vi "Intensity Graph to XY Graph.vi"() -> ()   [LabVIEW 2019]
uses:
  graph_utilities.lvclass
panel:
  in  "OK":bool
  out "Horizontal":cluster{dbl[], dbl[]}[](graph)
  out "Vertical":cluster{dbl[], dbl[]}[](graph)
  in  "V2f":dbl[][](graph)=array73x221[16133 elements]
  # "Control Graph:"
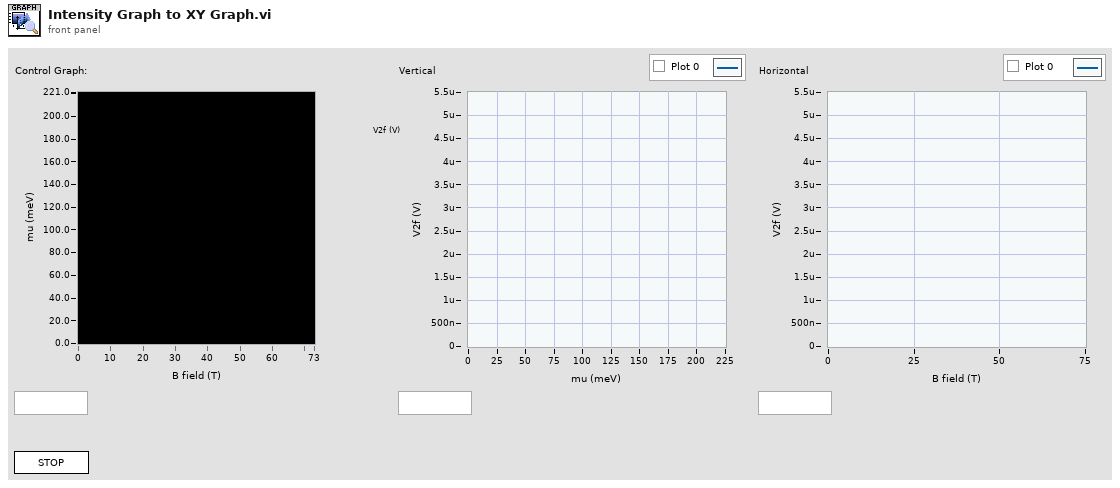
[diagram p1: front panel]
types:
  T1 = enum32{"Invalid", "Standard", "Closed", "Hidden", "Minimized", "Maximized"}
  T2 = enum32{"invalid app kind", "Development System", "Run Time System", "Student Edition", "Embedded LabVIEW", "Evaluation", "Custom"}
  T3 = cluster{"Core":cluster{"Current VI Reference":refnum<vi>, "Close Panel on Exit?":bool}, "graphs":refnum<class "graph_utilities.lvclass">[]}
  T4 = cluster{"Current VI Reference":refnum<vi>, "Close Panel on Exit?":bool}
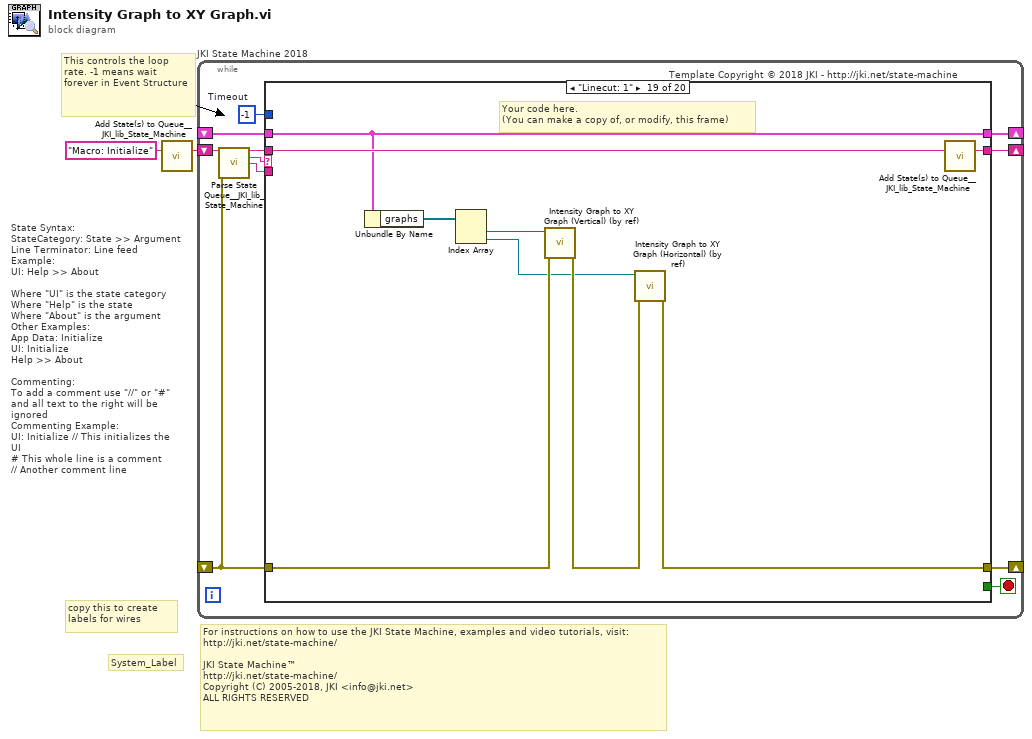
[diagram p0: block diagram]
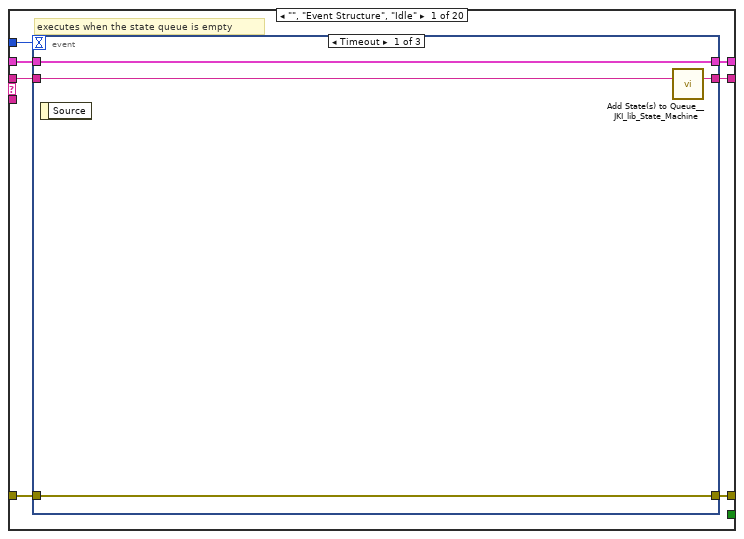
[diagram p2: hidden frame]
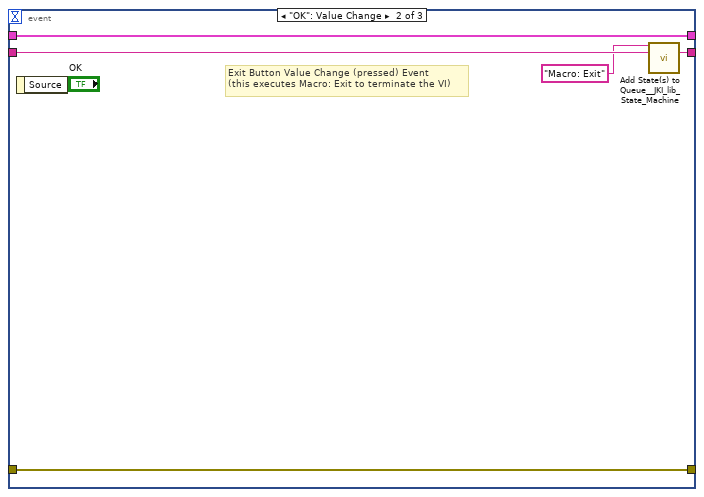
[diagram p3: hidden frame]
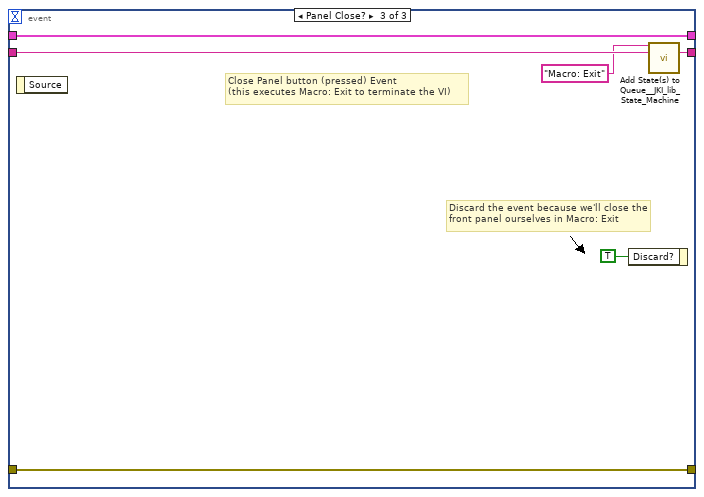
[diagram p4: hidden frame]
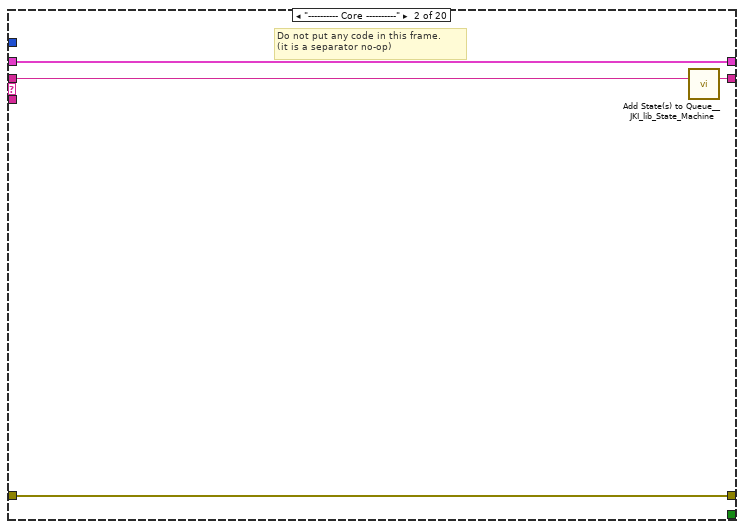
[diagram p5: hidden frame]
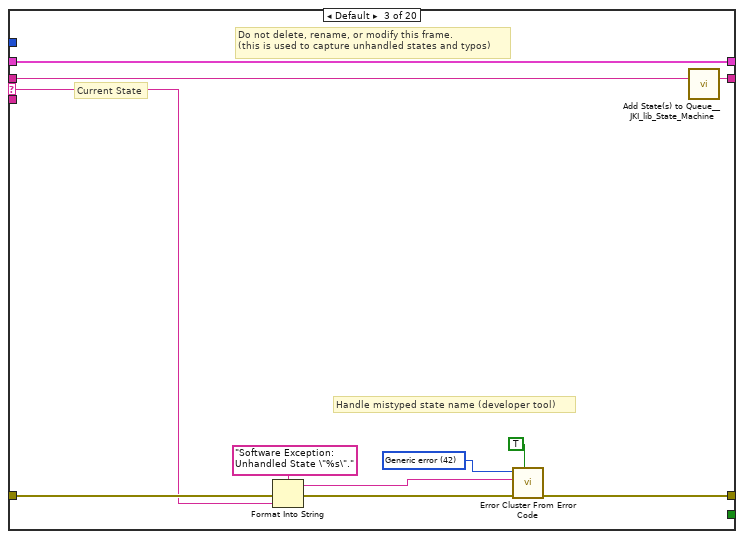
[diagram p6: hidden frame]
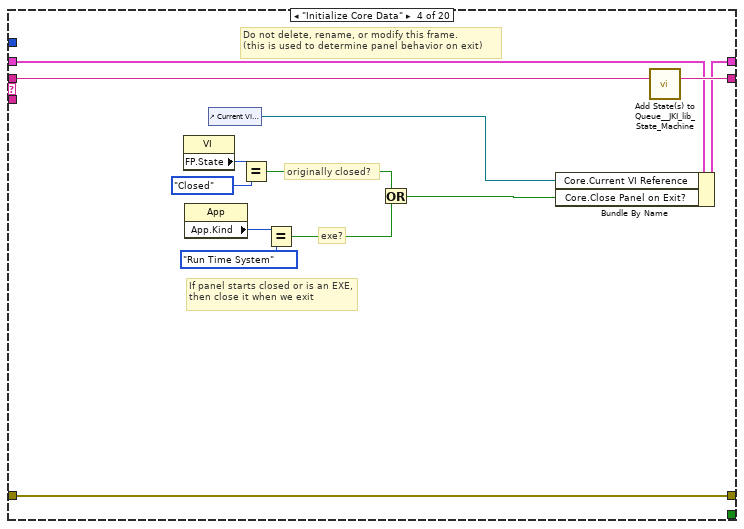
[diagram p7: hidden frame]
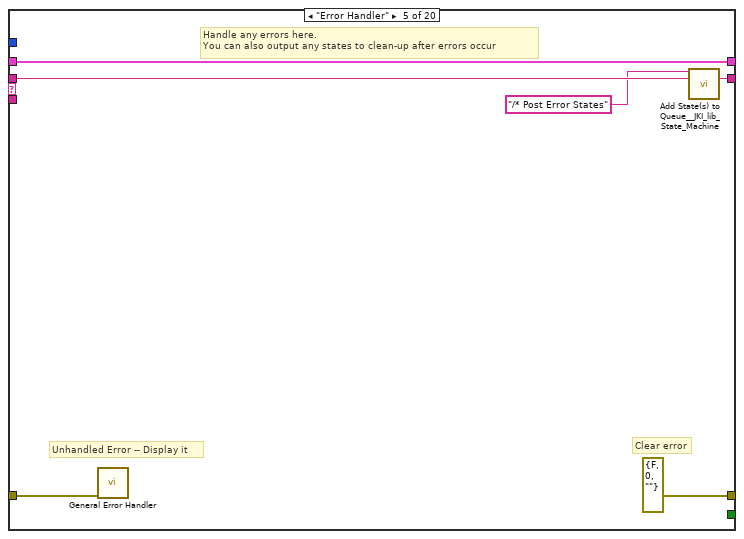
[diagram p8: hidden frame]
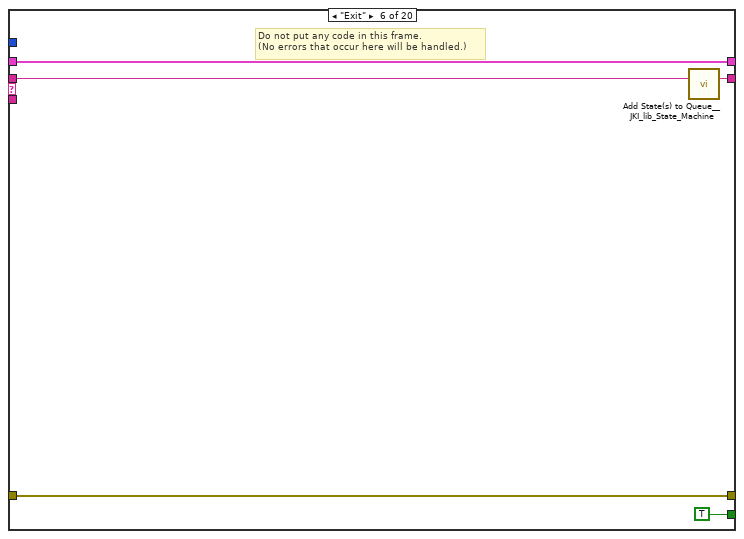
[diagram p9: hidden frame]
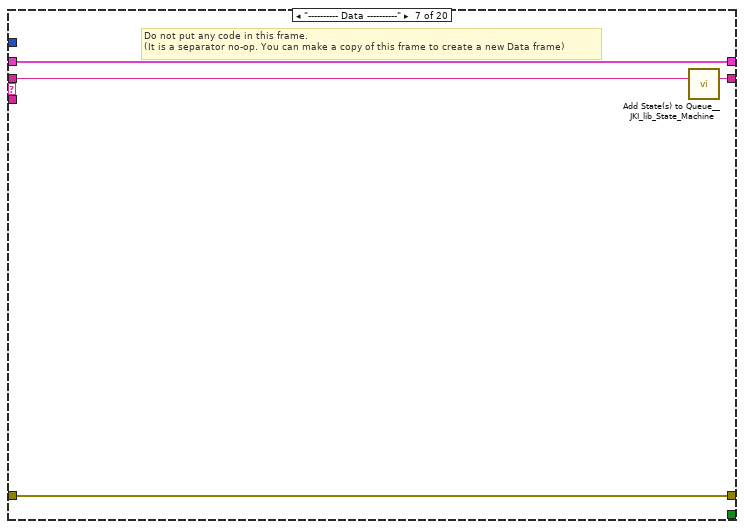
[diagram p10: hidden frame]
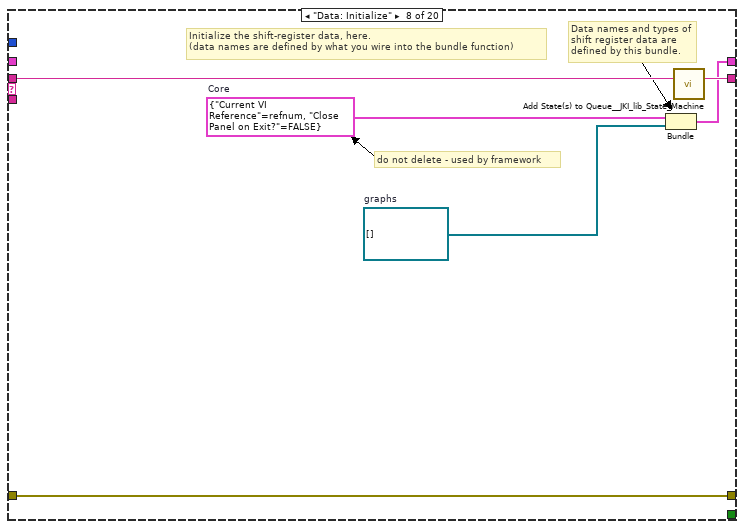
[diagram p11: hidden frame]
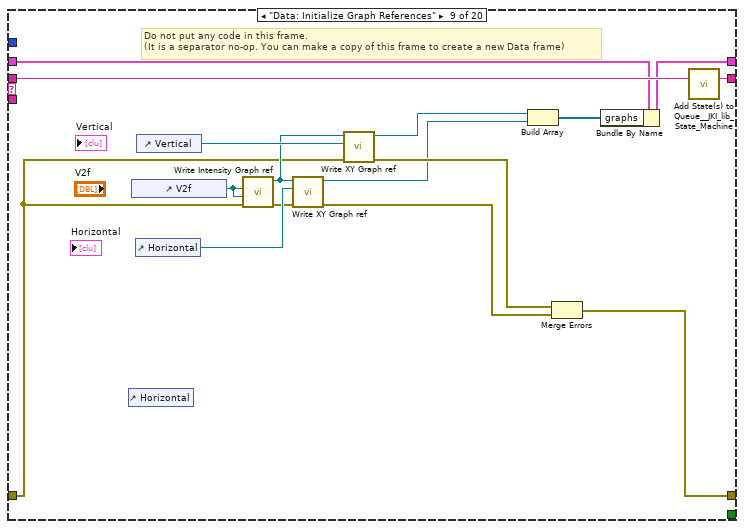
[diagram p12: hidden frame]
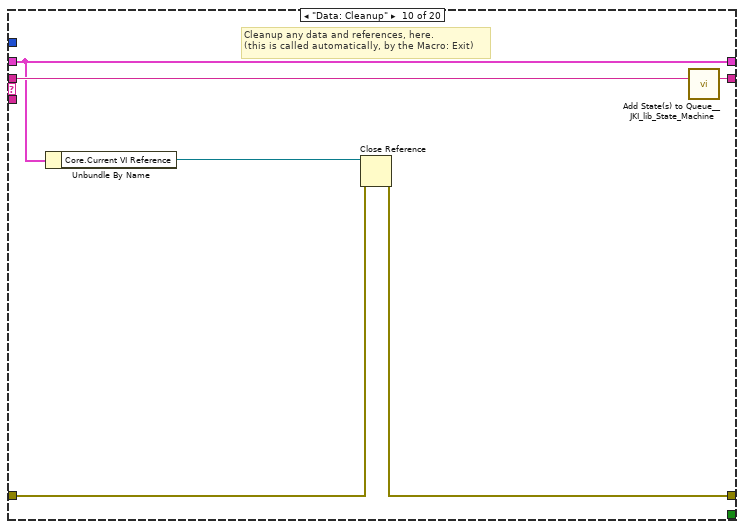
[diagram p13: hidden frame]
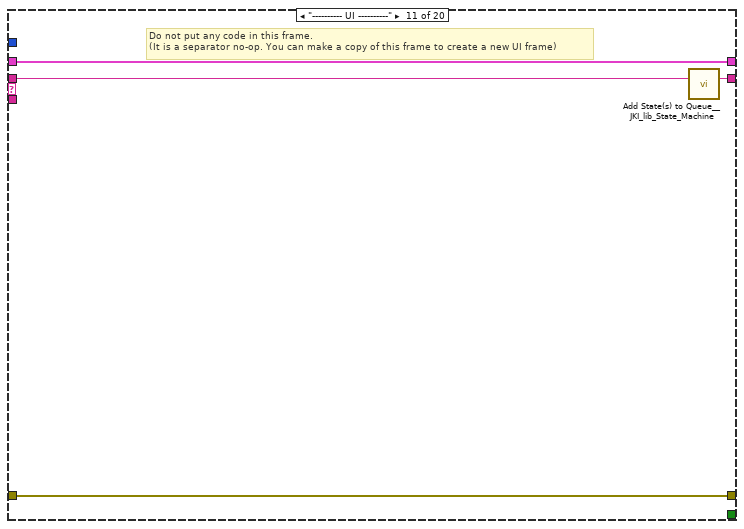
[diagram p14: hidden frame]
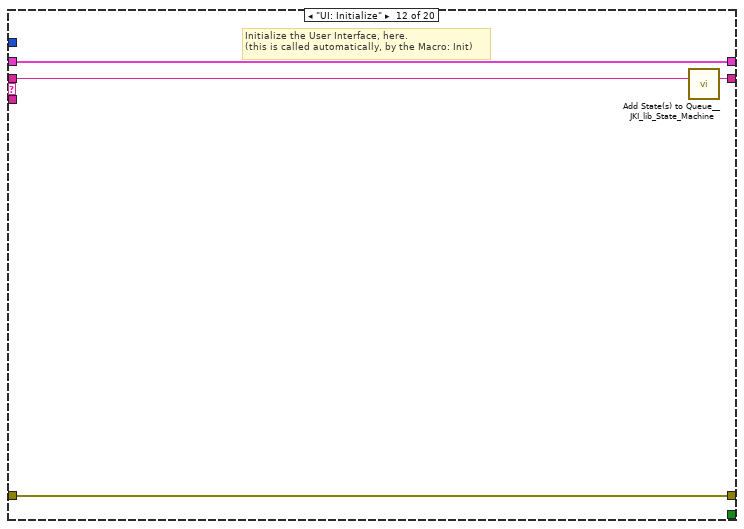
[diagram p15: hidden frame]
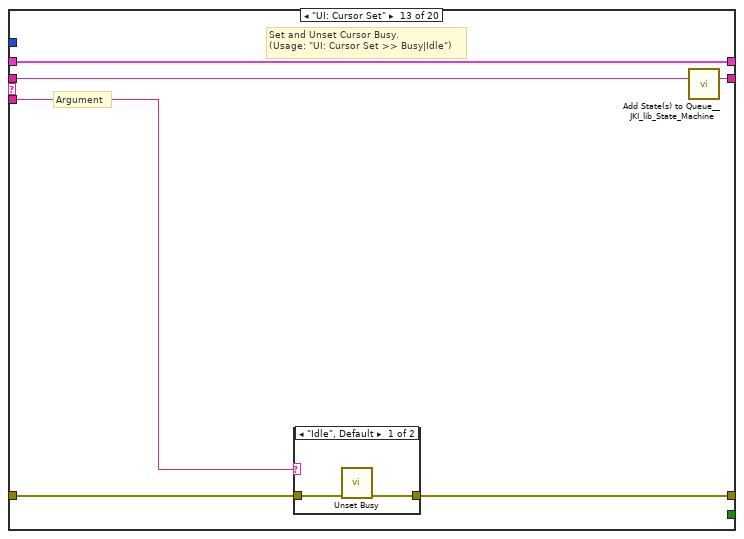
[diagram p16: hidden frame]
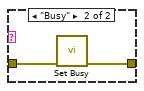
[diagram p17: hidden frame]
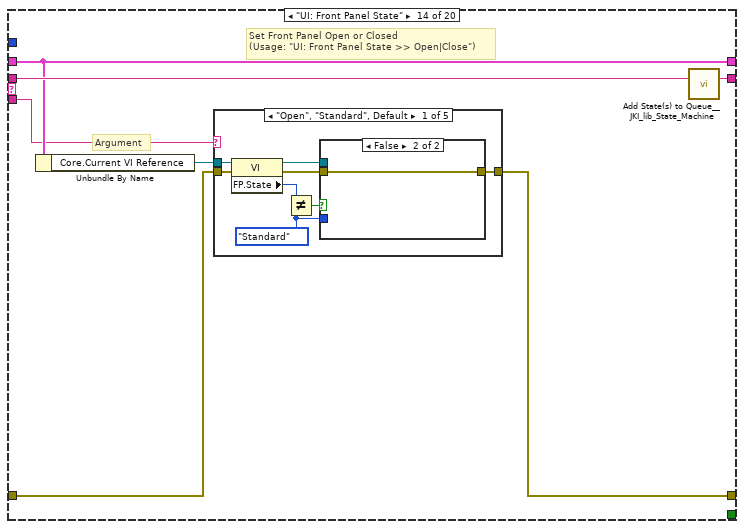
[diagram p18: hidden frame]
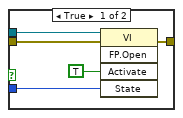
[diagram p19: hidden frame]
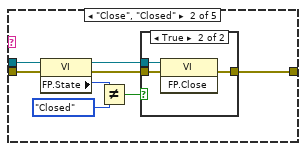
[diagram p20: hidden frame]
diagram:
  # "For instructions on how to use the JKI State Machine, examples and video tutorials, visit:\nhttp://jki.net/state-machine/\n\nJKI State Machine™\nhttp://jki.net/state-machine/\nCopyright (C) 2005-2018, JKI <info@jki.net>\nALL RIGHTS RESERVED"
  # "State Syntax:\nStateCategory: State >> Argument\nLine Terminator: Line feed\nExample:\nUI: Help >> About\n\nWhere \"UI\" is the state category\nWhere \"Help\" is the state\nWhere \"About\" is the argument\nOther Examples:\nApp Data: Initialize\nUI: Initialize\nHelp >> About\n\nCommenting:\nTo add a comment use \"//\" or \"#\" and all text to the right will be ignored\nCommenting Example:\nUI: Initialize // This initializes the UI\n# This whole line is a comment\n// Another comment line"
  # "copy this to create labels for wires"
  # "This controls the loop rate. -1 means wait forever in Event Structure"
  # "System_Label"
  n1 = call <vilib>:"Add State(s) to Queue__JKI_lib_State_Machine.vi"("State(s) in (\"\")"="Macro: Initialize") -> ("States Out"=w2:string)  [unwired: 14 in]
  n2 = while "JKI State Machine 2018" {
    shift-right: [w6] -> _
    shift-left: _ -> [w5]
    shift-right: [w9] -> _
    shift-left: _ -> [w3]
    shift-right: [w8] -> _
    shift-left: w2 -> [w10]
    stop <- w7 stop-if-true
    w4 = -1  # Timeout
    # "Template Copyright © 2018 JKI - http://jki.net/state-machine"
    n3 = call <vilib>:"Parse State Queue__JKI_lib_State_Machine.vi"("State Queue"=w10, "Error In (no error)"=w3) -> ("Remaining States"=w12:string, "Current State"=w13:string, "Arguments"=w11:string)  [unwired: 11 in]
    n4 = case shown="\"Linecut: 1\"" w13 {
      selector: w13 -> [_ _ w40 _ _ _ _ _ _ _ _ _ _ _ _ _ _ _ _ _]
      tunnel: w12 -> [w20 w39 w44 w63 w69 w74 w78 w84 w100 w106 w110 w114 w120 w131 w200 w206 w216 w220 w229 w233]
      tunnel: w11 -> [_ _ _ _ _ _ _ _ _ _ _ _ w115 w125 _ _ _ _ _ _]
      tunnel: w5 -> [w18 w36 w42 w56 w66 w72 w75 _ w91 w101 w107 w112 w118 w127 w197 w203 w213 w217 w227 w230]
      tunnel: [w17 w37 w46 w60 errorcluster {"status"=FALSE, "code"=0, "source"=""} ("error out") w71 w76 w81 w86 w102 w108 w111 w116 w128 w198 w204 w214 w218 w222 w231] -> w9
      tunnel: w3 -> [w16 w37 w45 w60 w65 w71 w76 w81 w85 w103 w108 w111 w117 w129 w198 w204 w214 w218 w224 w231]
      tunnel: [w19 w38 w43 w62 w68 w73 w77 w83 w99 w105 w109 w113 w119 w130 w199 w205 w215 w219 w228 w232] -> w8
      tunnel: [_ _ _ _ _ TRUE _ _ _ _ _ _ _ _ _ _ _ _ _ _] -> w7
      tunnel: [w15 w36 w42 w61 w66 w72 w75 w82 w90 w101 w107 w112 w118 w127 w197 w203 w213 w217 w227 w230] -> w6
      tunnel: w4 -> [w14 _ _ _ _ _ _ _ _ _ _ _ _ _ _ _ _ _ _ _]
      frame "", "Event Structure", "Idle" {
        # "executes when the state queue is empty"
        n5 = event shown="[0] Timeout" {
          selector: _ -> [_ _ _]
          dyn-events: _ -> [_ _ _]
          timeout: w14 -> [_ _ _]
          tunnel: w20 -> [w24 w29 w35]
          tunnel: [w23 w28 w34] -> w19
          tunnel: w18 -> [w21 w26 w32]
          tunnel: [w22 w27 w33] -> w17
          tunnel: w16 -> [w22 w27 w33]
          tunnel: [w21 w26 w32] -> w15
          event Timeout {
            n6 = event-data() -> ()  [unwired: 1 in, 1 out]
            n7 = call <vilib>:"Add State(s) to Queue__JKI_lib_State_Machine.vi"("State(s) in (\"\")"=w24) -> ("States Out"=w23:string)  [unwired: 14 in]
          }
          event "OK": Value Change {
            # "Exit Button Value Change (pressed) Event\n(this executes Macro: Exit to terminate the VI)"
            n8 = event-data() -> ()  [unwired: 1 in, 1 out]
            n9 = call <vilib>:"Add State(s) to Queue__JKI_lib_State_Machine.vi"("State(s) in Front (\"\")"="Macro: Exit", "State(s) in (\"\")"=w29) -> ("States Out"=w28:string)  [unwired: 13 in]
          }
          event Panel Close? {
            # "Discard the event because we'll close the front panel ourselves in Macro: Exit"
            # "Close Panel button (pressed) Event\n(this executes Macro: Exit to terminate the VI)"
            n10 = event-data() -> ()  [unwired: 1 in, 1 out]
            n11 = event-data("Discard?"=TRUE) -> ()  [unwired: 1 in, 1 out]
            n12 = call <vilib>:"Add State(s) to Queue__JKI_lib_State_Machine.vi"("State(s) in Front (\"\")"="Macro: Exit", "State(s) in (\"\")"=w35) -> ("States Out"=w34:string)  [unwired: 13 in]
          }
        }
      }
      frame "---------- Core ----------" {
        # "Do not put any code in this frame.\n(it is a separator no-op)"
        n13 = call <vilib>:"Add State(s) to Queue__JKI_lib_State_Machine.vi"("State(s) in (\"\")"=w39) -> ("States Out"=w38:string)  [unwired: 14 in]
      }
      frame Default {
        w49 = 42 items=["No error", "Argument error", "Memory is full", "Out of zone", "End of file", "File already open", "Generic file I/O error", "File not found", "File permission error", "Disk is full", "Duplicate path", "Too many files open", "System feature not enabled", "Resource file not found", "Cannot add resource", "Resource not found", "Image not found", "Image memory error", "Pen does not exist", "Config type invalid", "Config token not found", "Config parse error", "Config memory error", "Bad external code format", "Bad external code offset", "External code not present", "Null window", "Destroy window error", "Null menu", "Print aborted", "Bad print record", "Print driver error", "Windows error during printing", "Memory error during printing", "Print dialog error", "Generic print error", "Invalid device refnum", "Device not found", "Device parameter error", "Device unit error", "Cannot open device", "Device call aborted", "Generic error", "Cancelled by user", "Object ID too low", "Object ID too high", "Object not in heap", "Unknown heap", "Unknown object (invalid DefProc)", "Unknown object (DefProc not in table)", "Message out of range", "Invalid (null) method", "Unknown message", "Manager call not supported", "Bad address", "Network operation in progress", "Network operation timed out", "Connection is busy", "Network attribute not supported", "Network error", "Address in use", "System out of memory", "Connection aborted", "Connection refused", "Not connected", "Already connected", "Connection closed", "Initialization error (interapplication manager)", "Bad occurrence", "Wait on unbound occurrence handler", "Occurrence queue overflow", "Datalog type conflict", "Unused", "Unrecognized type (interapplication manager)", "Memory corrupt", "Failed to make temporary DLL", "Old CIN version", "Drag socket not found", "Failed to load drop-object", "Failed to register OLE object", "Failed to release OLE object", "Format specifier type mismatch", "Unknown format specifier", "Too few format specifiers", "Too many format specifiers", "Scan failed", "Newer CIN version", "Error converting to variant", "Runtime menu error", "Password tampered", "Variant attribute not found", "Incompatible variant data type", "Event data is not available", "Event Store is not present", "Occurrence is not found", "Event Queue is not created", "Event info is not available", "Refnum passed is NULL", "Error retrieving Class GUID", "Error retrieving CoClass GUID", "Error retrieving TypeLib GUID.", "Bad built application magic bytes.", "Specific driver is different from the specific driver associated with the Logical Name.", "There is no session opened to the class driver.", "Max Error", "MAX - Error with config objects", "MAX - Error loading configuration", "MAX - Group not supported"]
        # "Current State"
        # "Do not delete, rename, or modify this frame.\n(this is used to capture unhandled states and typos)"
        # "Handle mistyped state name (developer tool)"
        n14 = Format Into String(format string="Software Exception: Unhandled State \"%s\"." ("message"), error in=w45, w40) -> (resulting string=w48:string, error out=w47:errorcluster)  [unwired: 1 in]
        n15 = call <vilib>:"Error Cluster From Error Code.vi"("show call chain? (False)"=TRUE, "error in (no error)"=w47, "error message (\"\")"=w48, "error code (0)"=w49) -> ("error out"=w46:errorcluster)  [unwired: 5 in]
        n16 = call <vilib>:"Add State(s) to Queue__JKI_lib_State_Machine.vi"("State(s) in (\"\")"=w44) -> ("States Out"=w43:string)  [unwired: 14 in]
      }
      frame "Initialize Core Data" {
        # "Do not delete, rename, or modify this frame.\n(this is used to determine panel behavior on exit)"
        # "originally closed?"
        # "exe?"
        # "If panel starts closed or is an EXE, then close it when we exit"
        n17 = property class="VI"() -> ("FP.State"=w53:T1)  [unwired: 2 in, 2 out]
        n18 = property class="App"() -> ("App.Kind"=w59:T2)  [unwired: 2 in, 2 out]
        n19 = control-ref of="Current VI Reference"() -> (w54:refnum<vi>)
        n20 = Equal?(x=w53, y=T1."Closed" ("Front Panel Window:State")) -> (x = y?=w51:bool)
        n21 = Equal?(x=w59, y=T2."Run Time System" ("Application:Kind")) -> (x = y?=w57:bool)
        n22 = Or(x=w51, y=w57) -> (x .or. y?=w55:bool)
        n23 = Bundle By Name(cluster=w56, "Core.Current VI Reference"=w54, "Core.Close Panel on Exit?"=w55) -> (w61:T3)
        n24 = call <vilib>:"Add State(s) to Queue__JKI_lib_State_Machine.vi"("State(s) in (\"\")"=w63) -> ("States Out"=w62:string)  [unwired: 14 in]
      }
      frame "Error Handler" {
        # "Unhandled Error -- Display it"
        # "Handle any errors here.\nYou can also output any states to clean-up after errors occur"
        # "Clear error"
        n25 = call <vilib>:"General Error Handler.vi"("error in (no error)"=w65) -> ()  [unwired: 10 in, 5 out]
        n26 = call <vilib>:"Add State(s) to Queue__JKI_lib_State_Machine.vi"("State(s) in Front (\"\")"="/* Post Error States", "State(s) in (\"\")"=w69) -> ("States Out"=w68:string)  [unwired: 13 in]
      }
      frame "Exit" {
        # "Do not put any code in this frame.\n(No errors that occur here will be handled.)"
        n27 = call <vilib>:"Add State(s) to Queue__JKI_lib_State_Machine.vi"("State(s) in (\"\")"=w74) -> ("States Out"=w73:string)  [unwired: 14 in]
      }
      frame "---------- Data ----------" {
        # "Do not put any code in this frame.\n(It is a separator no-op. You can make a copy of this frame to create a new Data frame)"
        n28 = call <vilib>:"Add State(s) to Queue__JKI_lib_State_Machine.vi"("State(s) in (\"\")"=w78) -> ("States Out"=w77:string)  [unwired: 14 in]
      }
      frame "Data: Initialize" {
        w79 = refnum<class "graph_utilities.lvclass">[] []  # graphs
        w80 = T4 {"Current VI Reference"=refnum, "Close Panel on Exit?"=FALSE}  # Core
        # "do not delete - used by framework"
        # "Data names and types of shift register data are defined by this bundle."
        # "Initialize the shift-register data, here.\n(data names are defined by what you wire into the bundle function)"
        n29 = Bundle("Core"=w80, "graphs"=w79) -> (w82:T3)  [unwired: 1 in]
        n30 = call <vilib>:"Add State(s) to Queue__JKI_lib_State_Machine.vi"("State(s) in (\"\")"=w84) -> ("States Out"=w83:string)  [unwired: 14 in]
      }
      frame "Data: Initialize Graph References" {
        # "Do not put any code in this frame.\n(It is a separator no-op. You can make a copy of this frame to create a new Data frame)"
        n31 = control-ref of="Horizontal"() -> ()  [unwired: 1 out]
        n32 = control-ref of="V2f"() -> (w94:refnum<vi>)
        n33 = control-ref of="Horizontal"() -> (w96:refnum<vi>)
        n34 = control-ref of="Vertical"() -> (w98:refnum<vi>)
        n35 = call "Write Intensity Graph ref.vi"("error in (no error)"=w85, "Intensity Graph (Control)"=w94, "Intensity Graph"=w94) -> ("error out"=w95:errorcluster, "graph_utilities out"=w97:refnum<class "graph_utilities.lvclass">)  [unwired: 7 in]
        n36 = call "Write XY Graph ref.vi"("error in (no error)"=w95, "XY Graph"=w96, "graph_utilities in"=w97) -> ("error out"=w93:errorcluster, "graph_utilities out"=w88:refnum<class "graph_utilities.lvclass">)  [unwired: 7 in]
        n37 = call "Write XY Graph ref.vi"("error in (no error)"=w85, "XY Graph"=w98, "graph_utilities in"=w97) -> ("error out"=w92:errorcluster, "graph_utilities out"=w89:refnum<class "graph_utilities.lvclass">)  [unwired: 7 in]
        n38 = Build Array(w89, w88) -> (w87:refnum<class "graph_utilities.lvclass">[])
        n39 = Merge Errors(w92, w93) -> (w86:errorcluster)
        n40 = Bundle By Name(cluster=w91, "graphs"=w87) -> (w90:T3)
        n41 = call <vilib>:"Add State(s) to Queue__JKI_lib_State_Machine.vi"("State(s) in (\"\")"=w100) -> ("States Out"=w99:string)  [unwired: 14 in]
      }
      frame "Data: Cleanup" {
        # "Cleanup any data and references, here.\n(this is called automatically, by the Macro: Exit)"
        n42 = Unbundle By Name(w101) -> ("Core.Current VI Reference"=w104:refnum<vi>)
        n43 = Close Reference(reference=w104, error in (no error)=w103) -> (error out=w102:errorcluster)
        n44 = call <vilib>:"Add State(s) to Queue__JKI_lib_State_Machine.vi"("State(s) in (\"\")"=w106) -> ("States Out"=w105:string)  [unwired: 14 in]
      }
      frame "---------- UI ----------" {
        # "Do not put any code in this frame.\n(It is a separator no-op. You can make a copy of this frame to create a new UI frame)"
        n45 = call <vilib>:"Add State(s) to Queue__JKI_lib_State_Machine.vi"("State(s) in (\"\")"=w110) -> ("States Out"=w109:string)  [unwired: 14 in]
      }
      frame "UI: Initialize" {
        # "Initialize the User Interface, here.\n(this is called automatically, by the Macro: Init)"
        n46 = call <vilib>:"Add State(s) to Queue__JKI_lib_State_Machine.vi"("State(s) in (\"\")"=w114) -> ("States Out"=w113:string)  [unwired: 14 in]
      }
      frame "UI: Cursor Set" {
        # "Argument"
        # "Set and Unset Cursor Busy.\n(Usage: \"UI: Cursor Set >> Busy|Idle\")"
        n47 = case shown="\"Idle\", Default" w115 {
          tunnel: w117 -> [w122 w124]
          tunnel: [w121 w123] -> w116
          frame "Idle", Default {
            n48 = call <vilib>:"Unset Busy.vi"("error in (no error)"=w122) -> ("error out"=w121:errorcluster)  [unwired: 10 in]
          }
          frame "Busy" {
            n49 = call <vilib>:"Set Busy.vi"("error in (no error)"=w124) -> ("error out"=w123:errorcluster)  [unwired: 9 in, 1 out]
          }
        }
        n50 = call <vilib>:"Add State(s) to Queue__JKI_lib_State_Machine.vi"("State(s) in (\"\")"=w120) -> ("States Out"=w119:string)  [unwired: 14 in]
      }
      frame "UI: Front Panel State" {
        # "Argument"
        # "Set Front Panel Open or Closed\n(Usage: \"UI: Front Panel State >> Open|Close\")"
        n51 = Unbundle By Name(w127) -> ("Core.Current VI Reference"=w126:refnum<vi>)
        n52 = case shown="\"Open\", \"Standard\", Default" w125 {
          tunnel: w129 -> [w137 w152 w163 w176 w189]
          tunnel: [w139 w153 w165 w178 w191] -> w128
          tunnel: w126 -> [w138 w150 w164 w177 w190]
          frame "Open", "Standard", Default {
            w132 = T1."Standard" ("State")
            n53 = property class="VI"(reference=w138, error in=w137) -> (reference out=w135:refnum<vi>, error out=w136:errorcluster, "FP.State"=w134:T1)
            n54 = Not Equal?(x=w134, y=w132) -> (x != y?=w133:bool)
            n55 = case shown="False" w133 {
              tunnel: [w143 w145] -> w139
              tunnel: w136 -> [w142 w145]
              tunnel: w135 -> [w141 _]
              tunnel: w132 -> [w140 _]
              frame True {
                n56 = invoke class="VI" method="FP.Open"(reference=w141, error in=w142, "Activate"=TRUE, "State"=w140) -> (error out=w143:errorcluster)  [unwired: 1 in, 4 out]
              }
              frame False {
              }
            }
          }
          frame "Close", "Closed" {
            n57 = property class="VI"(reference=w150, error in=w152) -> (reference out=w149:refnum<vi>, error out=w151:errorcluster, "FP.State"=w147:T1)
            n58 = Not Equal?(x=w147, y=T1."Closed" ("Front Panel Window:State")) -> (x != y?=w146:bool)
            n59 = case shown="True" w146 {
              tunnel: [w154 w157] -> w153
              tunnel: w151 -> [w154 w156]
              tunnel: w149 -> [_ w155]
              frame False {
              }
              frame True {
                n60 = invoke class="VI" method="FP.Close"(reference=w155, error in=w156) -> (error out=w157:errorcluster)  [unwired: 1 in, 2 out]
              }
            }
          }
          frame "Hidden", "Hide" {
            w158 = T1."Hidden" ("State")
            n61 = property class="VI"(reference=w164, error in=w163) -> (reference out=w161:refnum<vi>, error out=w162:errorcluster, "FP.State"=w160:T1)
            n62 = Not Equal?(x=w160, y=w158) -> (x != y?=w159:bool)
            n63 = case shown="True" w159 {
              tunnel: [w169 w170] -> w165
              tunnel: w162 -> [w168 w170]
              tunnel: w161 -> [w167 _]
              tunnel: w158 -> [w166 _]
              frame True {
                n64 = invoke class="VI" method="FP.Open"(reference=w167, error in=w168, "State"=w166) -> (error out=w169:errorcluster)  [unwired: 2 in, 4 out]
              }
              frame False {
              }
            }
          }
          frame "Minimize", "Minimized" {
            w171 = T1."Minimized" ("State")
            n65 = property class="VI"(reference=w177, error in=w176) -> (reference out=w174:refnum<vi>, error out=w175:errorcluster, "FP.State"=w173:T1)
            n66 = Not Equal?(x=w173, y=w171) -> (x != y?=w172:bool)
            n67 = case shown="True" w172 {
              tunnel: [w182 w183] -> w178
              tunnel: w175 -> [w181 w183]
              tunnel: w174 -> [w180 _]
              tunnel: w171 -> [w179 _]
              frame True {
                n68 = invoke class="VI" method="FP.Open"(reference=w180, error in=w181, "State"=w179) -> (error out=w182:errorcluster)  [unwired: 2 in, 4 out]
              }
              frame False {
              }
            }
          }
          frame "Maximize", "Maximized" {
            w184 = T1."Maximized" ("State")
            n69 = property class="VI"(reference=w190, error in=w189) -> (reference out=w187:refnum<vi>, error out=w188:errorcluster, "FP.State"=w186:T1)
            n70 = Not Equal?(x=w186, y=w184) -> (x != y?=w185:bool)
            n71 = case shown="True" w185 {
              tunnel: [w195 w196] -> w191
              tunnel: w188 -> [w194 w196]
              tunnel: w187 -> [w193 _]
              tunnel: w184 -> [w192 _]
              frame True {
                n72 = invoke class="VI" method="FP.Open"(reference=w193, error in=w194, "State"=w192) -> (error out=w195:errorcluster)  [unwired: 2 in, 4 out]
              }
              frame False {
              }
            }
          }
        }
        n73 = call <vilib>:"Add State(s) to Queue__JKI_lib_State_Machine.vi"("State(s) in (\"\")"=w131) -> ("States Out"=w130:string)  [unwired: 14 in]
      }
      frame "---------- Macro ----------" {
        # "Do not put any code in this frame.\n(It is a separator no-op. You can make a copy of this frame to create a new Macro frame)"
        n74 = call <vilib>:"Add State(s) to Queue__JKI_lib_State_Machine.vi"("State(s) in (\"\")"=w200) -> ("States Out"=w199:string)  [unwired: 14 in]
      }
      frame "Macro: Initialize" {
        w202 = "Data: Initialize\nInitialize Core Data\nUI: Initialize\nUI: Front Panel State >> Open"  # Data: Initialize Initialize Core Data UI: Initialize UI: Front Panel State >> Open
        # "Initialization Macro\n(This is called once, when the VI starts)"
        n75 = call <vilib>:"Add State(s) to Queue__JKI_lib_State_Machine.vi"("State(s) in Front (\"\")"=w202, "State(s) in (\"\")"=w206, "State(s) at Back (\"\")"="Data: Initialize Graph References\nLinecut: 1\nMacro: Exit") -> ("States Out"=w205:string)  [unwired: 12 in]
      }
      frame "Macro: Exit" {
        # "Exit Macro\n(This is called once, when the VI exits)"
        n76 = Unbundle By Name(w213) -> ("Core.Close Panel on Exit?"=w212:bool)
        n77 = Select(t="UI: Front Panel State >> Close", s=w212, f="") -> (s? t:f=w209:string)
        n78 = call <vilib>:"Add State(s) to Queue__JKI_lib_State_Machine.vi"("State(s) in (\"\")"=w209, "State(s) at Back (\"\")"="Data: Cleanup\nExit") -> ("States Out"=w207:string)  [unwired: 13 in]
        n79 = call <vilib>:"Add State(s) to Queue__JKI_lib_State_Machine.vi"("State(s) in Front (\"\")"=w207, "State(s) in (\"\")"=w216) -> ("States Out"=w215:string)  [unwired: 13 in]
      }
      frame "---------- Linecut ----------" {
        # "Template Separator\n(You can make a copy of, or modify, this frame)"
        n80 = call <vilib>:"Add State(s) to Queue__JKI_lib_State_Machine.vi"("State(s) in (\"\")"=w220) -> ("States Out"=w219:string)  [unwired: 14 in]
      }
      frame "Linecut: 1" {
        # "Your code here.\n(You can make a copy of, or modify, this frame)"
        n81 = Unbundle By Name(w227) -> ("graphs"=w226:refnum<class "graph_utilities.lvclass">[])
        n82 = Index Array(array=w226) -> (element #1=w225:refnum<class "graph_utilities.lvclass">, element #2=w221:refnum<class "graph_utilities.lvclass">)  [unwired: 2 in]
        n83 = call "Intensity Graph to XY Graph (Vertical) (by ref).vi"("error in (no error)"=w224, "graph_utilities in"=w225) -> ("error out"=w223:errorcluster)  [unwired: 8 in, 1 out]
        n84 = call "Intensity Graph to XY Graph (Horizontal) (by ref).vi"("error in (no error)"=w223, "graph_utilities in"=w221) -> ("error out"=w222:errorcluster)  [unwired: 8 in, 1 out]
        n85 = call <vilib>:"Add State(s) to Queue__JKI_lib_State_Machine.vi"("State(s) in (\"\")"=w229) -> ("States Out"=w228:string)  [unwired: 14 in]
      }
      frame "Linecut: 2" {
        # "Your code here.\n(You can make a copy of, or modify, this frame)"
        n86 = call <vilib>:"Add State(s) to Queue__JKI_lib_State_Machine.vi"("State(s) in (\"\")"=w233) -> ("States Out"=w232:string)  [unwired: 14 in]
      }
    }
  }
